vi "Read Config.vi"(3 "error in (no error)":errorcluster) -> (7 "value":cluster{"Boolean Text":string, "Value":i32}[](array[cluster]), 10 "error out":errorcluster)   [LabVIEW 2020, in "Monedas.lvlib"]
uses:
  Monedas.lvlib
  <vilib>/Utility/xml.llb/Read From XML File(string).vi
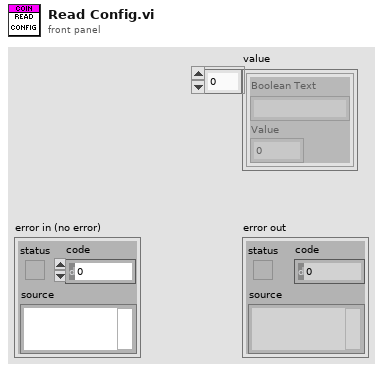
[diagram p1: front panel]
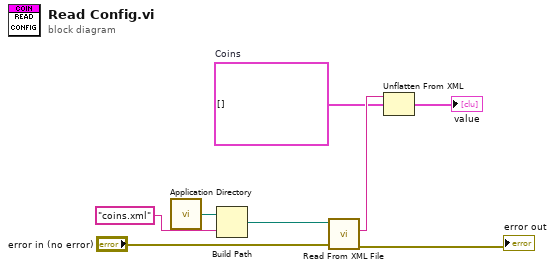
[diagram p0: block diagram]
diagram:
  w2 = cluster{"Boolean Text":string, "Value":i32}[] []  # Coins
  n1 = call <vilib>:"Application Directory.vi"() -> ("Application Directory"=w8:path)
  n2 = Build Path(base path=w8, name or relative path="coins.xml") -> (appended path=w6:path)
  n3 = call-poly <vilib>:"Read From XML File.vi"("error in (no error)"="error in (no error)", "XML File Path"=w6) -> ("error out"=→"error out":errorcluster, "XML Elements"=w3:string)  [unwired: 7 in, 1 out]
  n4 = Unflatten From XML(xml string=w3, type=w2) -> (value=→"value":cluster{"Boolean Text":string, "Value":i32}[])  [unwired: 1 in, 1 out]
